vi "SwerveDriveFace.vi"(0 "Strafe Joystick Axes":cluster{"X":dbl, "Y":dbl}, 1 "Face Joystick Axes":cluster{"X":dbl, "Y":dbl}, 3 "Face PID Gains":T2 {"derivative time (Td, min)" format="%.3f"; "integral time (Ti, min)" format="%.3f"; "proportional gain (Kc)" format="%.3f"}, 4 "Angle (degrees; 0 = right)":dbl, 5 "error in (no error)":errorcluster, 6 "Strafe Multiplier":dbl, 8 "Rotation Multiplier":dbl, 10 "Max Wheel Speed":dbl) -> (16 "Speed Chart":cluster{dbl, "Encoder Velocity":dbl}[](graph), 19 "error out":errorcluster)   [LabVIEW 2015]
uses:
  <vilib>/addons/control/pid/NI_PID_pid.lvlib
  <vilib>/addons/control/pid/pid.llb/PID Control Input Filter (DBL).vi
  <vilib>/addons/control/pid/pid.llb/PID (DBL).vi
  Team900SwerveDrive.lvlib
panel:
  out "diff.":dbl
  out "Waveform Chart":T1(graph)
  out "Robot Heading":dbl(knob) scale=3.1416..-3.1416
  out "Joystick Angle":dbl(knob) scale=3.1416..-3.1416
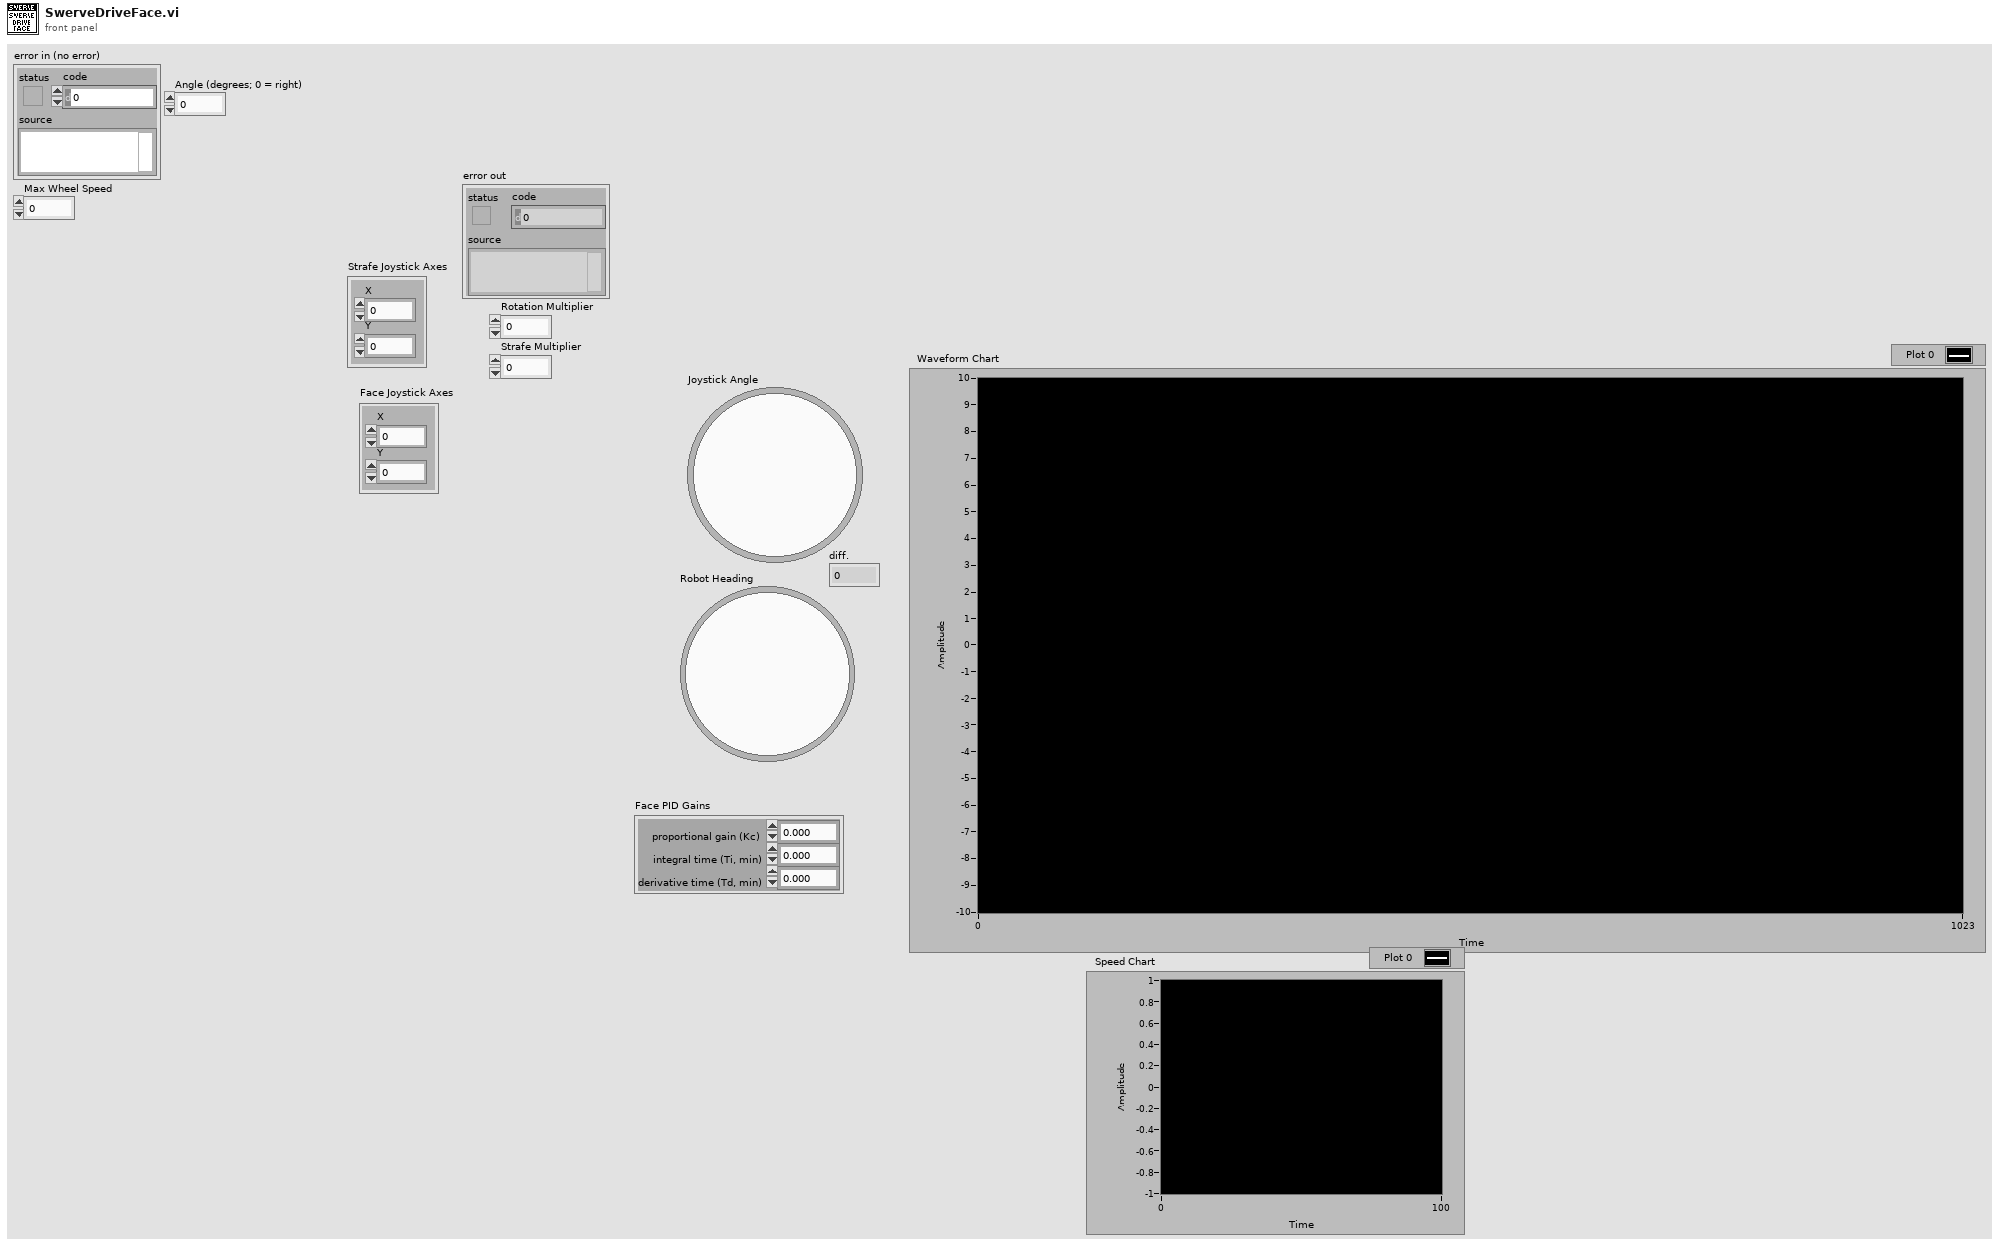
[diagram p1: front panel]
types:
  T1 = cluster{"output":dbl, "output":dbl, "millisecond timer value":u32}
  T2 = cluster{"proportional gain (Kc)":dbl, "integral time (Ti, min)":dbl, "derivative time (Td, min)":dbl}
  T3 = cluster{"output angle":dbl, "output":dbl, "millisecond timer value":u32}
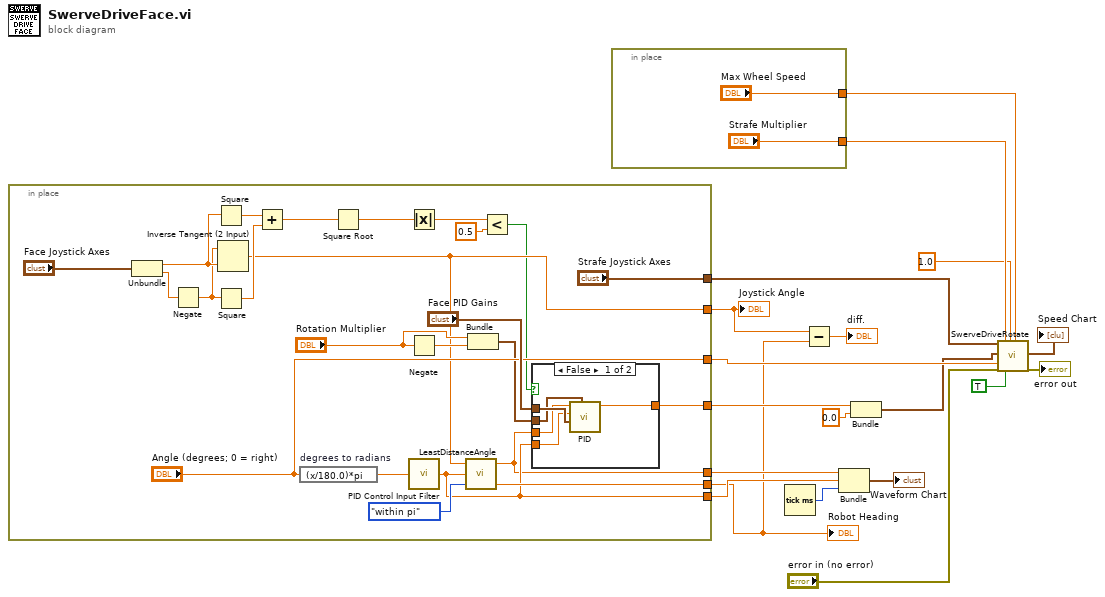
[diagram p0: block diagram]
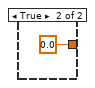
[diagram p2: hidden frame]
diagram:
  n1 = in-place {
    in-place-border: [w43] -> w17
    in-place-border: ["Strafe Joystick Axes"] -> w19
    in-place-border: ["Angle (degrees; 0 = right)"] -> w16
    in-place-border: [w23] -> w5
    in-place-border: [w25] -> w4
    in-place-border: [w21] -> w7
    in-place-border: [w20] -> w6
    n2 = Unbundle("Face Joystick Axes") -> ("X"=w35:dbl, "Y"=w34:dbl)
    n3 = Negate(x=w34) -> (-x=w29:dbl)
    n4 = Square(x=w35) -> (x^2=w39:dbl)
    n5 = Square(x=w29) -> (x^2=w38:dbl)
    n6 = Inverse Tangent (2 Input)(1:w35, 2:w29) -> (0:w23:dbl)
    n7 = Add(x=w39, y=w38) -> (x+y=w37:dbl)
    n8 = expression code="(x/180.0)*pi" "degrees to radians"("Angle (degrees; 0 = right)") -> (w40:dbl)
    n9 = Square Root(x=w37) -> (sqrt(x)=w36:dbl)
    n10 = Absolute Value(x=w36) -> (abs(x)=w32:dbl)
    n11 = Negate(x="Rotation Multiplier") -> (-x=w27:dbl)
    n12 = call-poly <vilib>:"PID Control Input Filter.vi"("input"=w40) -> ("output"=w21:dbl)  [unwired: 4 in]
    n13 = call "LeastDistanceAngle.vi"("Enum"=enum16{"within pi", "within pi/2"}."within pi", "Current angle"=w21, "target angle (between pi and -pi) 2"=w23) -> ("current angle (between pi and -pi) 2"=w25:dbl, "output angle"=w20:dbl)  [unwired: 1 out]
    n14 = Bundle("Rotation Multiplier"="Rotation Multiplier", w27) -> (w26:cluster{"Rotation Multiplier":dbl, dbl})  [unwired: 1 in]
    n15 = Less?(x=w32, y=0.5) -> (x < y?=w22:bool)
    n16 = case shown="False" w22 {
      tunnel: [w48 0.0 ("output")] -> w43
      tunnel: "Face PID Gains" -> [w47 _]
      tunnel: w26 -> [w46 _]
      tunnel: w21 -> [w45 _]
      tunnel: w20 -> [w44 _]
      frame False {
        n17 = call-poly <vilib>:"PID.vi"("output range"=w46, "PID gains"=w47, "process variable"=w45, "setpoint"=w44) -> ("output"=w48:dbl)  [unwired: 6 in, 1 out]
      }
      frame True {
      }
    }
  }
  "Joystick Angle" <- w5
  "Robot Heading" <- w4
  n18 = in-place {
    in-place-border: ["Max Wheel Speed"] -> w12
    in-place-border: ["Strafe Multiplier"] -> w9
  }
  n19 = Tick Count (ms)() -> (millisecond timer value=w11:u32)
  n20 = Subtract(x=w5, y=w4) -> (x-y=→"diff.":dbl)
  n21 = Bundle("output angle"=w6, "output"=w7, "millisecond timer value"=w11) -> (→"Waveform Chart":T3)  [unwired: 1 in]
  n22 = Bundle("output"=w17, 0.0) -> (w2:cluster{"output":dbl, dbl})  [unwired: 1 in]
  n23 = call "SwerveDriveRotate.vi"("Strafe Joystick Axes"=w19, "Trigger Axes"=w2, "Angle (degrees; 0 = right)"=w16, "error in (no error)"="error in (no error)", "Strafe Multiplier"=w9, "FieldCentric? (T)"=TRUE, "Rotation Multiplier"=1.0, "Max Wheel Speed"=w12) -> ("Speed Chart"=→"Speed Chart":cluster{dbl, "Encoder Velocity":dbl}[], "error out"=→"error out":errorcluster)  [unwired: 9 in, 1 out]
